vi "MBUS_U16toString.vi"(10 "Format":u16(ring) items=["Decimal", "Hexadecimal", "String"], 11 "U16_in":u16[](array[numeric])) -> (3 "String_out":string)   [LabVIEW 2012, in "MBUS_Modbus.lvlib"]
uses:
  MBUS_Modbus.lvlib
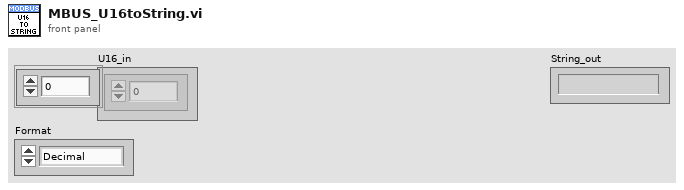
[diagram p1: front panel]
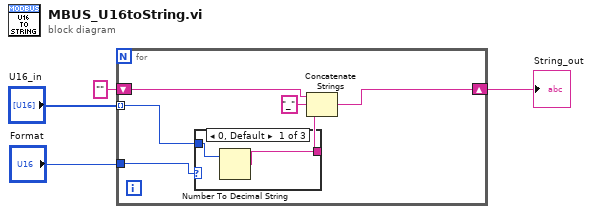
[diagram p0: block diagram]
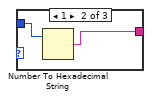
[diagram p2: hidden frame]
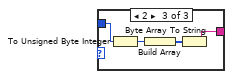
[diagram p3: hidden frame]
diagram:
  n1 = for {
    tunnel: "U16_in" -> [w10] mode=indexing
    shift-right: [w6] -> w3
    shift-left: "" -> [w7]
    tunnel: "Format" -> [w5]
    n2 = case shown="0, Default" w5 {
      tunnel: w10 -> [w12 w14 w18]
      tunnel: [w11 w13 w17] -> w9
      frame 0, Default {
        n3 = Number To Decimal String(number=w12) -> (decimal integer string=w11:string)  [unwired: 1 in]
      }
      frame 1 {
        n4 = Number To Hexadecimal String(2:w14) -> (0:w13:string)  [unwired: 1 in]
      }
      frame 2 {
        n5 = To Unsigned Byte Integer(number=w18) -> (unsigned 8bit integer=w16:u8)
        n6 = Build Array(w16) -> (w15:u8[])
        n7 = Byte Array To String(unsigned byte array=w15) -> (string=w17:string)
      }
    }
    n8 = Concatenate Strings(w7, "_" ("string"), w9) -> (w6:string)
  }
  "String_out" <- w3
